vi "GenerateExcelHeader.vi"(10 "Number of Columns":u64, 11 "Number of Rows":u64) -> (3 "Excel Header":string)   [LabVIEW 2014]
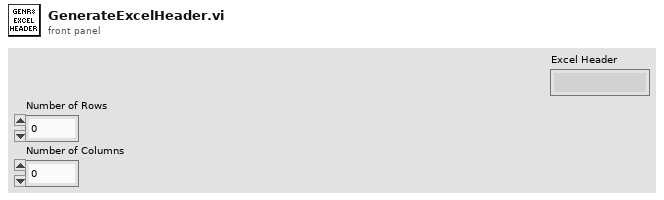
[diagram p1: front panel]
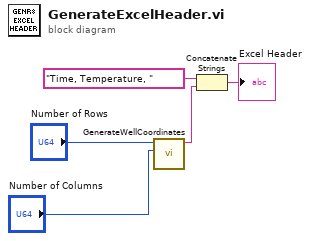
[diagram p0: block diagram]
diagram:
  n1 = call "GenerateWellCoordinates.vi"("Columns"="Number of Columns", "Rows"="Number of Rows") -> ("Well Coordinates"=w1:string)  [unwired: 9 in]
  n2 = Concatenate Strings("Time, Temperature, ", w1) -> (→"Excel Header":string)
